vi "TurnOn.vi"(7 "Voltage Set (V)":dbl, 8 "error in (no error)":errorcluster, 9 "OCP Level (A)":dbl, 10 "OVP Level (V)":dbl, 11 "PSU_N87 in":refnum<class "PSU_N67.lvclass">) -> (0 "error out":errorcluster, 3 "PSU_N87 out":refnum<class "PSU_N67.lvclass">)   [LabVIEW 2014, in "PSU_N67.lvclass"]
uses:
  PSU_N67.lvclass
  PSU.lvclass/PSU.ctl
  PSU_N67.lvclass/PSU_N67.ctl
  Read Channel.vi
  PSU.lvclass
  <instrlib>/Agilent N6700 Series/Agilent N6700 Series.lvlib
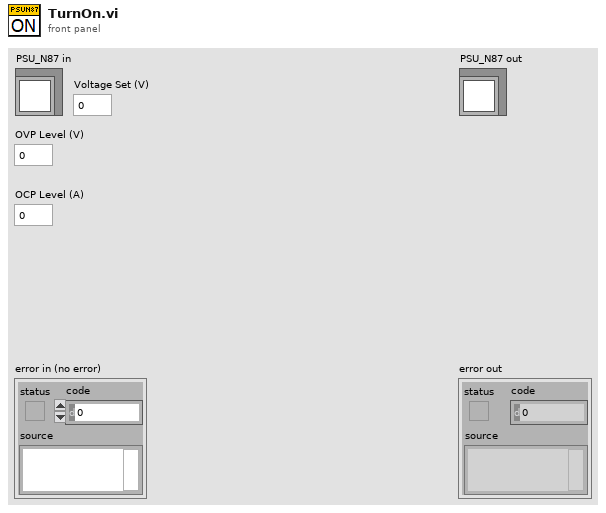
[diagram p1: front panel]
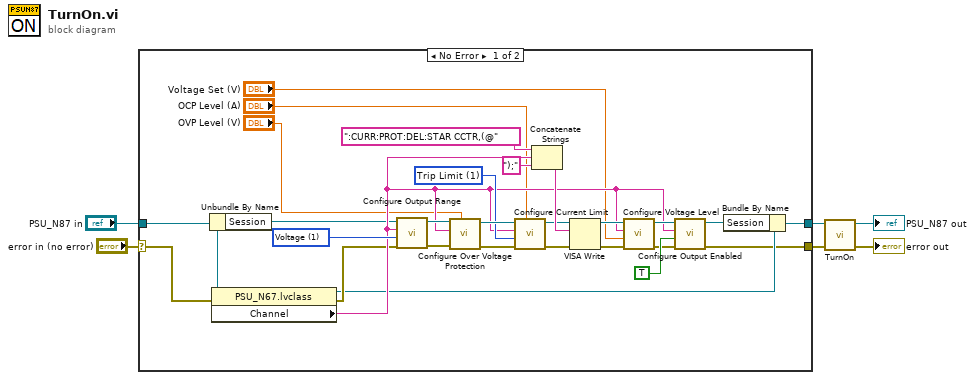
[diagram p0: block diagram]
diagram:
  n1 = case shown="No Error" "error in (no error)" {
    selector: "error in (no error)" -> [w16 w36]
    tunnel: [w9 w36] -> w3
    tunnel: "PSU_N87 in" -> [w18 w35]
    tunnel: [w13 w35] -> w4
    frame No Error {
      w23 = 1 items=["Regulatory Limit", "Trip Limit"] ("Behavior (0: Regulatory Limit)")
      w19 = 1 items=["Voltage"=1, "Current"=0] ("Range Type (1: Voltage)")
      n2 = Unbundle By Name(w18) -> ("Session"=w7:refnum<visa-resource-name>)
      n3 = property class="PSU_N67.lvclass"(reference=w18, error in=w16) -> (reference out=w12:refnum<class "PSU_N67.lvclass">, error out=w15:errorcluster, "Channel"=w17:string)
      n4 = call <instrlib>:"Configure Output Range.vi"("error in (no error)"=w15, "Range Type (1: Voltage)"=w19, "Channel Name (1)"=w17, "VISA resource name"=w7) -> ("error out"=w25:errorcluster, "VISA resource name out"=w24:refnum<visa-resource-name>)  [unwired: 6 in]
      n5 = call <instrlib>:"Configure Over Voltage Protection.vi"("Limit (0.0 volts)"="OVP Level (V)", "error in (no error)"=w25, "Channel Name (1)"=w17, "VISA resource name"=w24) -> ("error out"=w27:errorcluster, "VISA resource name out"=w26:refnum<visa-resource-name>)  [unwired: 6 in]
      n6 = call <instrlib>:"Configure Current Limit.vi"("Limit (0.0 amps)"="OCP Level (A)", "error in (no error)"=w27, "Behavior (0: Regulatory Limit)"=w23, "Channel Name (1)"=w17, "VISA resource name"=w26) -> ("error out"=w29:errorcluster, "VISA resource name out"=w28:refnum<visa-resource-name>)  [unwired: 5 in]
      n7 = Concatenate Strings(":CURR:PROT:DEL:STAR CCTR,(@" ("format string"), w17, ");" ("string")) -> (w34:string)
      n8 = VISA Write(VISA resource name=w28, write buffer=w34, error in (no error)=w29) -> (VISA resource name out=w30:refnum<visa-resource-name>, error out=w31:errorcluster)  [unwired: 1 out]
      n9 = call <instrlib>:"Configure Voltage Level.vi"("error in (no error)"=w31, "Level  (0.0 volts)"="Voltage Set (V)", "Channel Name (1)"=w17, "VISA resource name"=w30) -> ("error out"=w20:errorcluster, "VISA resource name out"=w21:refnum<visa-resource-name>)  [unwired: 6 in]
      n10 = call <instrlib>:"Configure Output Enabled.vi"("error in (no error)"=w20, "Enable Output (False)"=TRUE, "Channel Name (1)"=w17, "VISA resource name"=w21) -> ("error out"=w9:errorcluster, "VISA resource name out"=w14:refnum<visa-resource-name>)  [unwired: 6 in]
      n11 = Bundle By Name(cluster=w12, "Session"=w14) -> (w13:refnum<class "PSU_N67.lvclass">)
    }
    frame Error {
    }
  }
  n12 = call-parent "TurnOn.vi"("error in (no error)"=w3, "PSU in"=w4) -> ("error out"=→"error out":errorcluster, "PSU out"=→"PSU_N87 out":refnum<class "PSU_N67.lvclass">)  [unwired: 8 in]
